vi "ReadConfiguration_DataArray.vi"(8 "error in (no error)":errorcluster, 11 "VI Path":path=path "D:/") -> (0 "error out":errorcluster, 3 "DataArray":cluster{"Data name":string, "Data":variant}[](array[cluster]))   [LabVIEW 2015]
uses:
  <vilib>/Utility/config.llb/Read Key (String).vi
  <vilib>/Utility/config.llb/NI_LVConfig.lvlib
panel:
  out "Secetion Array":string[][](array[string])
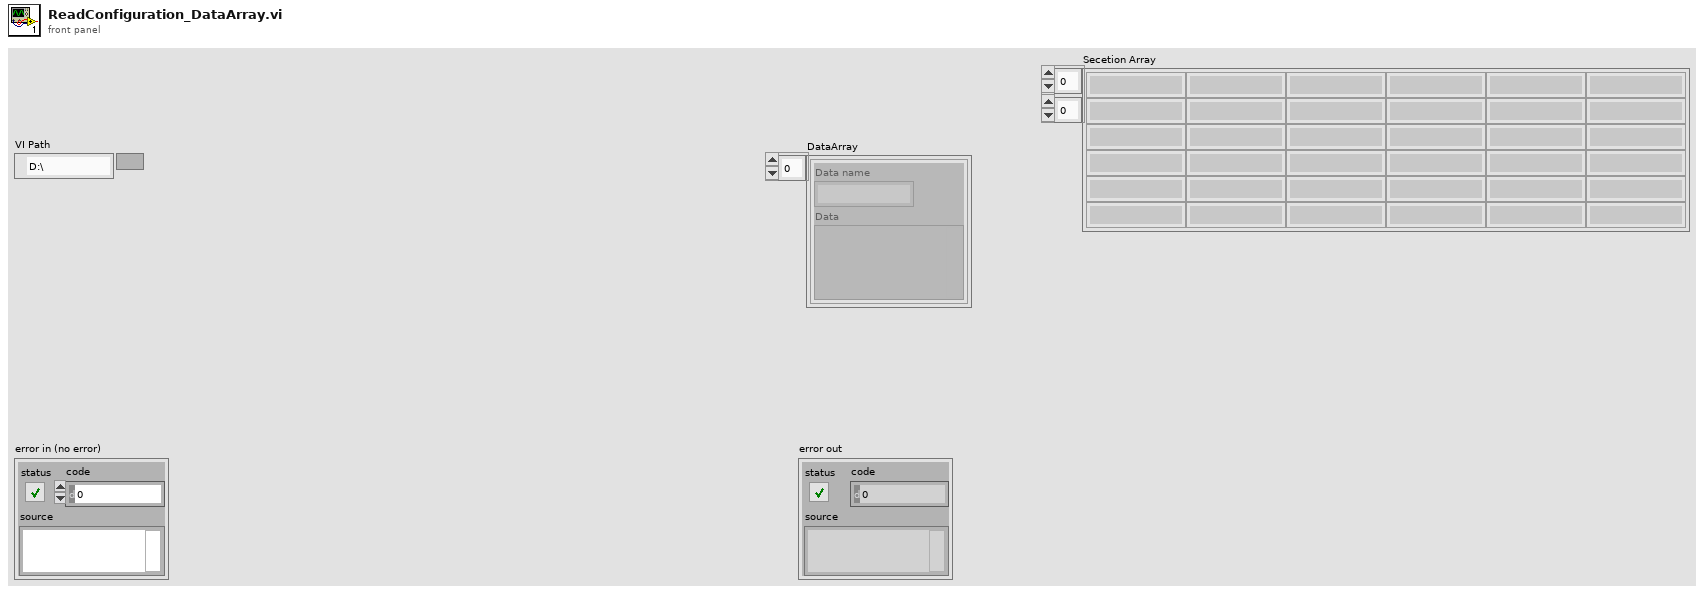
[diagram p1: front panel]
types:
  T1 = typedef "NI_LVConfig.lvlib/Config Data RefNum.ctl" = refnum<k1>
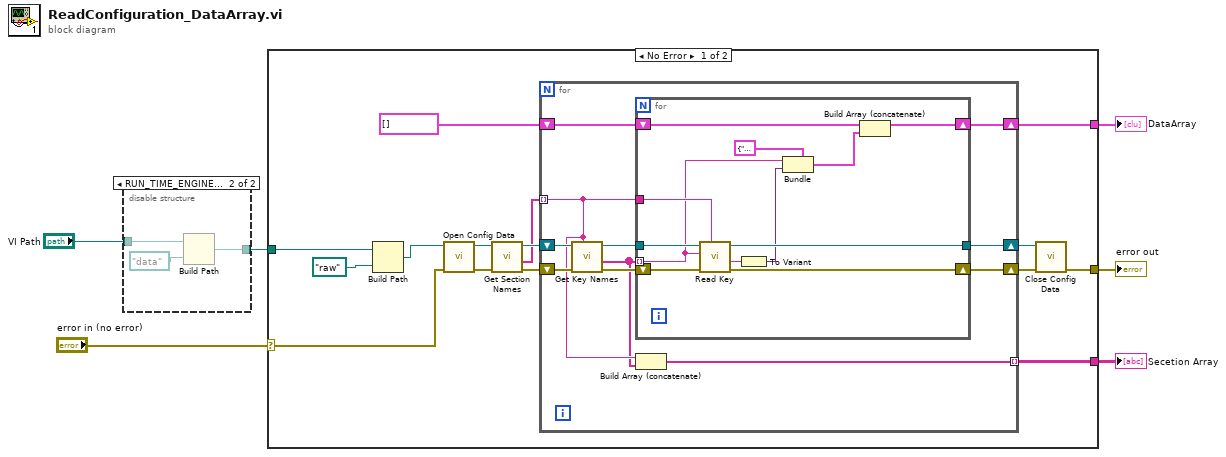
[diagram p0: block diagram]
diagram:
  n1 = disable-structure shown="RUN_TIME_ENGINE==True" {
    disable-tunnel: "VI Path" -> [w7 w10]
    disable-tunnel: [w7 w9] -> w3
    frame condition #0 (active) {
    }
    frame condition #1 {
      n2 = Build Path(base path=w10, name or relative path=path "data") -> (appended path=w9:path)
    }
  }
  n3 = case shown="No Error" "error in (no error)" {
    selector: "error in (no error)" -> [w24 w49]
    tunnel: [w25 w49] -> w5
    tunnel: w3 -> [w17 _]
    tunnel: [w14 _] -> w2
    tunnel: [w11 _] -> w1
    frame No Error {
      n4 = Build Path(base path=w17, name or relative path=path "raw") -> (appended path=w15:path)
      n5 = call <vilib>:"Open Config Data.vi"("error in (no error)"=w24, "configuration file path"=w15) -> ("error out"=w19:errorcluster, "refnum"=w21:T1)  [unwired: 7 in, 1 out]
      n6 = call <vilib>:"Get Section Names.vi"("error in (no error)"=w19, "refnum"=w21) -> ("error out"=w18:errorcluster, "section names"=w12:string[], "refnum out"=w20:T1)  [unwired: 7 in]
      n7 = for {
        shift-right: [w34] -> w22
        shift-left: w20 -> [w32]
        shift-right: [w36] -> w23
        shift-left: w18 -> [w31]
        tunnel: w12 -> [w28] mode=indexing
        shift-right: [w30] -> w14
        shift-left: cluster{"Data name":string, "Data":variant}[] [] -> [w29]
        tunnel: [w26] -> w11 mode=indexing
        n8 = call <vilib>:"Get Key Names.vi"("section"=w28, "error in (no error)"=w31, "refnum"=w32) -> ("error out"=w35:errorcluster, "key names"=w27:string[], "refnum out"=w33:T1)  [unwired: 5 in, 1 out]
        n9 = for {
          tunnel: w33 -> [w48]
          tunnel: w28 -> [w47]
          shift-right: [w46] -> w36
          shift-left: w35 -> [w45]
          tunnel: w27 -> [w42] mode=indexing
          tunnel: [w44] -> w34
          shift-right: [w37] -> w30
          shift-left: w29 -> [w38]
          n10 = call-poly <vilib>:"Read Key.vi"("section"=w47, "error in (no error)"=w45, "key"=w42, "refnum"=w48) -> ("error out"=w46:errorcluster, "value"=w43:string, "refnum out"=w44:T1)  [unwired: 4 in, 1 out]
          n11 = To Variant(anything=w43) -> (Variant=w41:variant)
          n12 = Bundle(cluster=cluster{"Data name":string, "Data":variant} {"Data name"="", "Data"=variant} ("Data  Out"), "Data name"=w42, "Data"=w41) -> (w39:cluster{"Data name":string, "Data":variant})
          n13 = Build Array (concatenate)(w38, w39) -> (w37:cluster{"Data name":string, "Data":variant}[])
        }
        n14 = Build Array (concatenate)(w28, w27) -> (w26:string[])
      }
      n15 = call <vilib>:"Close Config Data.vi"("error in (no error)"=w23, "refnum"=w22) -> ("error out"=w25:errorcluster)  [unwired: 8 in, 1 out]
    }
    frame Error {
    }
  }
  "error out" <- w5
  "DataArray" <- w2
  "Secetion Array" <- w1
